vi "NI6071E.ReadDB.vi"(0 "i ref in":refnum<vi>, 5 "error in":errorcluster) -> (14 "i ref out":refnum<vi>, 19 "error out":errorcluster)   [LabVIEW 2014, in "NI6071E.lvlib"]
doc: "This vi reads out the database entry and stores the relevant data to the object's attributes."
uses:
  NI6071E.lvlib
  CSCore/BaseProcess/BaseProcess.lvlib
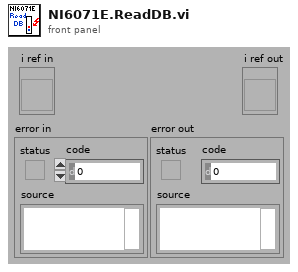
[diagram p1: front panel]
types:
  T1 = typedef "BaseProcess.lvlib/BaseProcess.i attribute.ctl" = cluster{"EventStatus":string, "EventError":i32, "PresetEvtWatchD":i32, "PresetPdcWatchD":i32, "EventTimeout":i32, "PeriodicInterval":i32, "Interface":string[], "Address":string[], "Special":string[], "PeriodicError":i32, "PeriodicStatus":string, "SuperProc":string, "Descriptors":T2[], "CaseRef":refnum<vi>, "PdcRef":refnum<vi>, "Thread Ref":refnum<vi>, "eventErrorID":i32, "eventStatusID":i32, "periodicErrorID":i32, "periodicStatusID":i32, "pdcCtrID":i32}
  T2 = typedef "BaseProcess.lvlib/BaseProcess.descriptor definition.ctl" = cluster{"selector":string, "descriptor":T3}
  T3 = typedef "BaseProcess.lvlib/BaseProcess.descriptor string definition.ctl" = string
  T4 = typedef "NI6071E.lvlib/NI6071E.i attribute.ctl" = cluster{"NI6071E Server":string, "Port":u16, "NI6071E Config":T5, "NI6071E Start":T6, "Waveforms":waveform(dbl)[], "RT Error":errorcluster, "NI6071E Read":T7, "connection ID":refnum<k5>, "DAQ Status":string, "device (1)":i16, "DAQ Status Service ID":i32}
  T5 = typedef "NI6071E.lvlib/NI6071EConfig.ctl" = cluster{"device (1)":i16, "channels (0)":tag[], "buffer size (1000 scans)":i32, "[number of buffers] (1)":i32, "measurement mode structure":cluster{"measurement mode":u16, "reserved":u32}, "input limits (no change)":cluster{"high limit (0.0)":sgl, "low limit (0.0)":sgl}[], "coupling & input config (no change:0)":cluster{"coupling (no change:0)":enum16{"no change", "DC", "AC", "GND", "internal ref."}, "input config (no change:0)":u16}[]}
  T6 = typedef "NI6071E.lvlib/NI6071EStart.ctl" = cluster{"scan rate (40000 scans/sec)":sgl, "trigger type (analog)":enum16{"no trigger", "analog", "digital A", "digital A & B", "scan clock gate"}, "edge or slope \n(rising)":enum16{"no change", "rising", "falling"}, "number of buffers to acquire (1)":i32, "analog chan (PFI0) & level (2.00)":cluster{"trigger channel (empty)":string, "level (0.0)":sgl}, "[additional trig params]":cluster{"hysteresis (0.0)":sgl, "coupling (no change:0)":enum16{"no change", "DC", "AC"}, "delay (0 sec)":sgl, "skip count (0)":i32, "time limit (0 sec)":sgl}}
  T7 = typedef "NI6071E.lvlib/NI6071ERead.ctl" = cluster{"time limit in sec (-1:auto calculate)":sgl, "number of scans to read (-1:all)":i32}
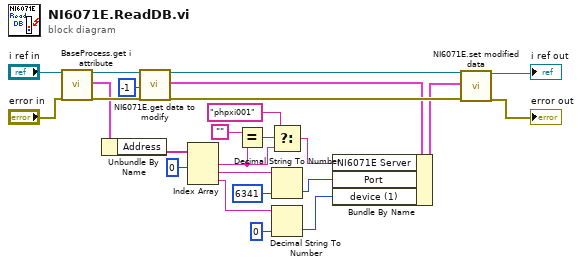
[diagram p0: block diagram]
diagram:
  n1 = call "BaseProcess.get i attribute.vi"("i ref in"="i ref in", "error in (no error)"="error in") -> ("i ref out"=w22:refnum<vi>, "i attribute"=w1:T1, "error out"=w23:errorcluster)  [unwired: 15 in]
  n2 = Unbundle By Name(w1) -> ("Address"=w2:string[])
  n3 = call "NI6071E.get data to modify.vi"("i ref in"=w22, "ms timeout (-1)"=-1, "error in (no error)"=w23) -> ("i ref out"=w18:refnum<vi>, "i attribute"=w5:T4, "error out"=w19:errorcluster)  [unwired: 13 in, 1 out]
  n4 = Index Array(array=w2, index #1=0 ("index")) -> (element #1=w10:string, element #2=w7:string, element #3=w16:string)  [unwired: 2 in]
  n5 = Equal?(x="", y=w10) -> (x = y?=w9:bool)
  n6 = Select(t="phpxi001", s=w9, f=w10) -> (s? t:f=w11:string)
  n7 = Decimal String To Number(string=w7, default (0L)=6341 ("default (0 I32)")) -> (number=w6:i32)  [unwired: 1 in, 1 out]
  n8 = Decimal String To Number(string=w16, default (0L)=0 ("default (0 I32)")) -> (number=w15:i32)  [unwired: 1 in, 1 out]
  n9 = Bundle By Name(cluster=w5, "NI6071E Server"=w11, "Port"=w6, "device (1)"=w15) -> (w13:T4)
  n10 = call "NI6071E.set modified data.vi"("i ref in"=w18, "i attribute"=w13, "error in (no error)"=w19) -> ("i ref out"=→"i ref out":refnum<vi>, "error out"=→"error out":errorcluster)  [unwired: 15 in]
